vi "GyroGet.vi"(0 "refnum name":string="My I2C RefNum") -> (14 "xdot":dbl format="%.2f", 15 "ydot":dbl, 16 "zdot":dbl format="%.2f", 17 "x":dbl, 18 "y":dbl, 19 "z":dbl)   [LabVIEW 2014]
panel:
  out "ztemp":dbl
  out "ytemp":dbl
  out "xtemp":dbl
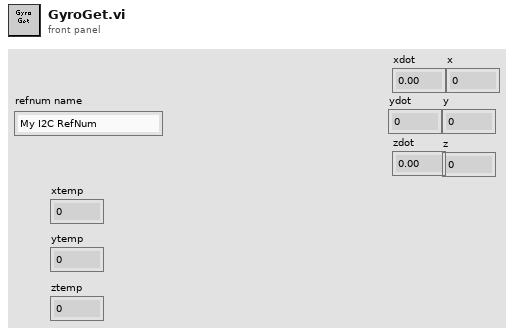
[diagram p1: front panel]
types:
  T1 = typedef "WPI_I2CDevRef.ctl" = cluster{"DevStatus":errorcluster, "Controller":T2, "Device Address":u8, "Handle":i32, "I2C Bus":T3}
  T2 = typedef "FPGA_TypedefDigitalModule.ctl" = enum16{"Controller 1"}
  T3 = typedef "i2c_bus.ctl" = enum16{"I2C On-Board", "I2C MXP", "Invalid"}
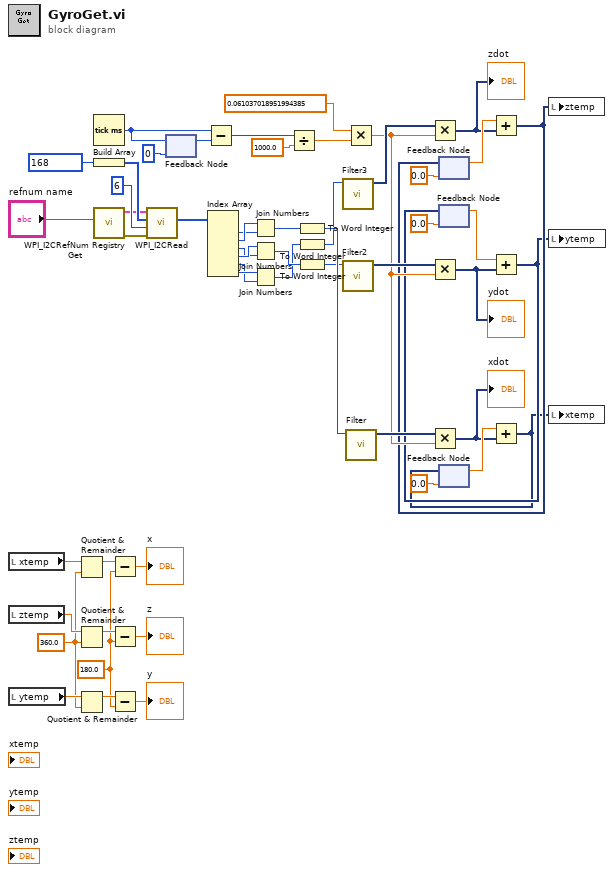
[diagram p0: block diagram]
diagram:
  w4 = 180.0 ("y")
  w8 = 360.0 ("y")
  n1 = local read "xtemp"() -> (w9:dbl)
  n2 = local read "ztemp"() -> (w11:dbl)
  n3 = local read "ytemp"() -> (w10:dbl)
  n4 = Quotient & Remainder(x=w9, y=w8) -> (x-y*floor(x/y)=w5:dbl)  [unwired: 1 out]
  n5 = Quotient & Remainder(x=w11, y=w8) -> (x-y*floor(x/y)=w7:dbl)  [unwired: 1 out]
  n6 = Quotient & Remainder(x=w10, y=w8) -> (x-y*floor(x/y)=w6:dbl)  [unwired: 1 out]
  n7 = Tick Count (ms)() -> (millisecond timer value=w20:u32)
  n8 = Build Array(u8 168) -> (w52:u8[])
  n9 = call <vilib>:"WPI_I2CRefNum Registry Get.vi"("refnum name"="refnum name") -> ("error out"=w38:errorcluster, "I2CDevRef"=w39:T1)  [unwired: 9 in]
  n10 = Subtract(x=w5, y=w4) -> (x-y=→"x":dbl)
  n11 = Subtract(x=w7, y=w4) -> (x-y=→"z":dbl)
  n12 = Subtract(x=w6, y=w4) -> (x-y=→"y":dbl)
  n13 = call <vilib>:"WPI_I2CRead.vi"("error in (no error)"=w38, "I2CBytesToRead"=u8 6, "I2CRegister"=w52, "I2CDevRef"=w39) -> ("Data Out"=w50:u8[])  [unwired: 5 in, 2 out]
  n14 = feedback-in #1(w20) -> ()
  n15 = feedback #1(u32 0 ("millisecond timer value")) -> (w21:u32)
  n16 = Subtract(x=w20, y=w21) -> (x-y=w18:u32)
  n17 = Index Array(array=w50) -> (element #1=w48:u8, element #2=w49:u8, element #3=w46:u8, element #4=w47:u8, element #5=w44:u8, element #6=w45:u8)  [unwired: 6 in]
  n18 = Join Numbers(hi=w49, lo=w48) -> ((hi.lo)=w43:u16)
  n19 = Join Numbers(hi=w47, lo=w46) -> ((hi.lo)=w42:u16)
  n20 = Join Numbers(hi=w45, lo=w44) -> ((hi.lo)=w41:u16)
  n21 = Divide(x=w18, y=1000.0) -> (x/y=w16:dbl)
  n22 = To Word Integer(number=w43) -> (16bit integer=w37:i16)
  n23 = To Word Integer(number=w41) -> (16bit integer=w36:i16)
  n24 = To Word Integer(number=w42) -> (16bit integer=w35:i16)
  n25 = call "Filter3"("Signal"=w36) -> ("Filtered Signal"=w24:dynamicdata)  [unwired: 9 in, 1 out]
  n26 = call "Filter2"("Signal"=w35) -> ("Filtered Signal"=w28:dynamicdata)  [unwired: 9 in, 1 out]
  n27 = Multiply(x=0.061037018951994385 ("y"), y=w16) -> (x*y=w15:dbl)
  n28 = call "Filter"("Signal"=w37) -> ("Filtered Signal"=w26:dynamicdata)  [unwired: 9 in, 1 out]
  n29 = Multiply(x=w24, y=w15) -> (x*y=w23:dynamicdata)
  "zdot" <- w23
  n30 = Multiply(x=w28, y=w15) -> (x*y=w27:dynamicdata)
  "ydot" <- w27
  n31 = Multiply(x=w26, y=w15) -> (x*y=w25:dynamicdata)
  "xdot" <- w25
  n32 = feedback #2(0.0) -> (w29:dbl)
  n33 = feedback #3(0.0) -> (w31:dbl)
  n34 = feedback #4(0.0) -> (w30:dbl)
  n35 = Add(x=w29, y=w23) -> (x+y=w14:dynamicdata)
  n36 = feedback-in #2(w14) -> ()
  n37 = Add(x=w31, y=w27) -> (x+y=w13:dynamicdata)
  n38 = feedback-in #3(w13) -> ()
  n39 = Add(x=w30, y=w25) -> (x+y=w12:dynamicdata)
  n40 = feedback-in #4(w12) -> ()
  n41 = local write "ztemp"(w14) -> ()
  n42 = local write "ytemp"(w13) -> ()
  n43 = local write "xtemp"(w12) -> ()
